vi "Terminate.vi"(8 "error in (no error)":errorcluster, 10 "Message in":refnum<class "TerminateMessage.lvclass">, 11 "LineCCD in":refnum<class "LineCCD.lvclass">) -> (0 "error out":errorcluster, 3 "LineCCD out":refnum<class "LineCCD.lvclass">)   [LabVIEW 2012, in "LineCCD.lvclass"]
doc: "This member function is called when the statemachine in the run.vi receives an 'terminate' command. It closes the RabbitMQ connection. \n\nOverride this member function in your derived class to release all previously acquired resources (but don't forget to call the parent method). If your component has subcomponents, they count as resources, and you have to release them by calling their own terminate functions."
uses:
  LineCCD.lvclass
  <vilib>/Distrio/Murmex/Murmex/Murmex.lvclass
  <instrlib>/ALPHALAS CCD S Series/ALPHALAS CCD S Series.lvlib
  <vilib>/Distrio/Murmex/TerminateMessage/TerminateMessage.lvclass
panel:
  # "This method is called when the TERMINATE\ntrigger is sent. \n\nOverride this method when your component needs to\nrespond to this trigger. \n\nCall parent for proper implementation"
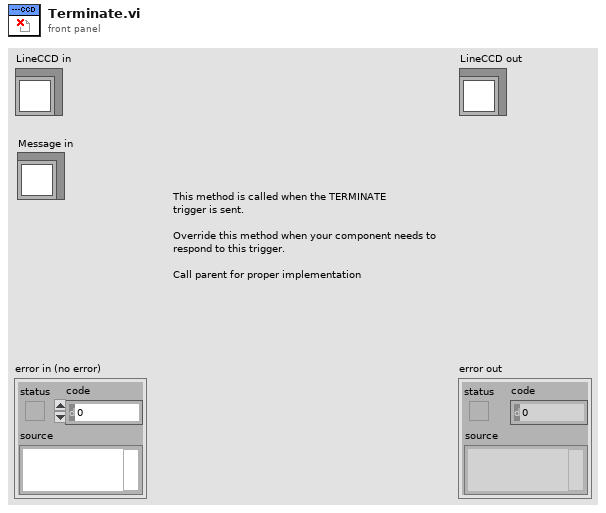
[diagram p1: front panel]
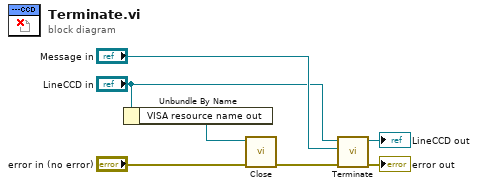
[diagram p0: block diagram]
diagram:
  n1 = Unbundle By Name("LineCCD in") -> ("VISA resource name out"=w1:refnum<visa-resource-name>)
  n2 = call <instrlib>:"Close.vi"("error in (no error)"="error in (no error)", "VISA resource name"=w1) -> ("error out"=w3:errorcluster)  [unwired: 9 in]
  n3 = call-parent "Terminate.vi"("error in (no error)"=w3, "Message in"="Message in", "Murmex in"="LineCCD in") -> ("error out"=→"error out":errorcluster, "Murmex out"=→"LineCCD out":refnum<class "LineCCD.lvclass">)  [unwired: 7 in]
